vi "Leviathan_Main_v4.1.0.vi"() -> ()   [LabVIEW 2025]
doc: "In that day, the Lord will punish with his sword - his fierce, great and powerful sword - Leviathan the gliding serpent, Leviathan the coiling serpent; he will slay the monster of the sea.\n-Isaiah 27:1"
uses:
  <vilib>/DAQmx/read.llb/DAQmx Read (Analog 2D DBL NChan NSamp).vi
  94cf692e-9ffa-4bb0-948f-941e7388c268.vi
  9a7535df-366d-4375-9b4f-c4f5a7296935.vi
  <vilib>/DAQmx/write.llb/DAQmx Write (Analog 1D Wfm NChan NSamp).vi
  89056647-3b37-41a7-a948-164930831248.vi
  <vilib>/DAQmx/miscellaneous.llb/DAQmx Fill In Error Info.vi
panel:
  out "Femto Gain V/A":dbl
  in  "Femto Gain V/A":dbl(ring) items=["1E3"=1.0, "1E4"=2.0, "1E5"=3.0, "1E6"=4.0, "1E7"=5.0, "1E8"=6.0, "1E9"=7.0]
  in  "Ch Swap Delay / ms":dbl=50.0 format="%0.0f"
  in  "RESET":bool
  out "# saved":i32
  out "Piezo V":dbl format="%_5g"
  out "Crashed?":bool
  out "G / G0":dbl
  in  "PID ON?":bool
  out "OffGuide":dbl(graph)
  in  "Reset2D":bool
  in  "Reset1D":bool
  in  "RT Analysis ON?":bool
  in  "SAVE?":bool
  out "2D Hist":dbl[][](graph)
  out "RT Bias num / V":dbl
  out "RT Femto num / V":dbl format="%#_3g"
  out "Piezo (V)":dbl(slide) scale=-7.0..7.0
  out "Hist":i32[](graph)
  out "Log(G/G0)":dbl[](graph)
  out "RT Signal":T1(graph)
  in  "Selector":T2(tab)
  in  "PID gains":T3={"proportional gain (Kc)"=-0.01, "integral time (Ti, min)"=9.999999999999982e-05, "derivative time (Td, min)"=0.0} {"derivative time (Td, min)" format="%.6f"; "integral time (Ti, min)" format="%.6f"; "proportional gain (Kc)" format="%.6f"}
  in  "SP Femto / V":dbl=0.1
  out "PID Runtime / s":dbl
  in  "Pulse Bias / V":dbl
  in  "PM wave shape":dbl(ring) items=["triangle", "square", "sine"]
  in  "PM amplitude / nm":dbl
  in  "No of Piezo Modulations per step":dbl
  out "Ramp Time / s":dbl
  in  "Ramp?":bool
  in  "Rp Hgt":dbl=10.0 caption="Ramp Height / nm"
  in  "Ramp Time (1) /s":dbl=1.0
  in  "Offset (0) / nm":dbl min=-200.0 max=200.0 step=1.0 format="%.1g"
  in  "Ramp Select":u16(ring) caption="Ramp Type" items=["Linear Ramp", "Advanced Ramps"]
  in  "Exp Typ":u16(ring) caption="Adv BJ Measurement Method" items=["Piezo Hold", "Square Bias", "Sine Bias", "Triangle Bias", "IV", "PM", "IV - Polarity Sweep", "CV - 2 Terminal", "Pre/Post Pulse IVs WIP"]
  in  "Bias Amp / V":dbl=1.0 caption="Bias Amplitude / V"
  in  "dZ / nm":dbl=1.0 caption="Step Height / nm"
  in  "Steps":i32=10 caption="No of Steps"
  in  "Bias f / Hz":dbl=100.0 caption="Bias modulation frequency / Hz"
  in  "Modulation hold time (0.01) / s":dbl=0.01
  in  "Sharpening Time /s (1) /s":dbl=1.0
  in  "sharpening depth /nm":dbl=50.0
  in  "#Traces/Sharpen":i32=200
  in  "Minimum Log(G/G0)":dbl=-6.0
  in  "Minimum Piezo / nm":dbl=-0.25
  in  "Maximum Log(G/G0)":dbl=0.5
  in  "Maximum Piezo / nm":dbl=3.2
  in  "Upper Bound":dbl=0.5
  in  "Lower Bound":dbl=-5.0
  in  "G0 alignement":dbl=-0.5
  in  "2DHist Intensity":dbl(slide)=101.26582278481013 scale=0.0..3000.0
  out "Ramps":dbl[][](graph)
  in  "Offset (0) / 1E-5":dbl
  in  "Piezo Sensitivity / nm V-1":dbl=1.95
  in  "File Path":path
  in  "Aq Rt (20000) / Hz":dbl=20000.0 format="%0.0f"
  out "Acquire":bool
  in  "DC Bias (0.2) / V":dbl=0.2 format="%_4g"
  # "Leviathan v4.1.0\nJames M. F. Morris | R. Tom Abram | Chiara E. Spano | Roberto Listo | Adam Larbi | Zoë Irlam | Andrea Vezzoli"
  # "Controls:\n\nPg Up - increase offset by 1nm\nHome - Decrease offset by 1 nm\nInsert - Start/Stop Saving\nDelete - Start/Stop PID\nEnd - Start/Stop Ramp\nPg Down - Start/Stop Real time analysis\n\nSaving formatting change:\nDO NOT include a file extension when choosing a \nfile name (e.g. use Directory\\James\\SaveFile NOT Directory\\James\\SaveFile.txt)\n\nPID Info:\nTurning the PID off and leaving the Ramp engaged will activate manual ('James')\nmode.\n\nNOTES:\nThe RESET buttons have a bug, they need to be held down for them to work. Working on fixing this."
  # "NOTES:\n\nPIEZO OSCILATION SETTINGS:\nOscilation frequency calculation:\n\nHold Time = Ramp time / No of steps (units: seconds)\nT  = Hold Time - DC Time (units: seconds)\nOscilation Frequency = No of Piezo Modulations / T (units: hertz)\n\nOscilation amplitude = 2 * PM amplitude (units: nanometers)"
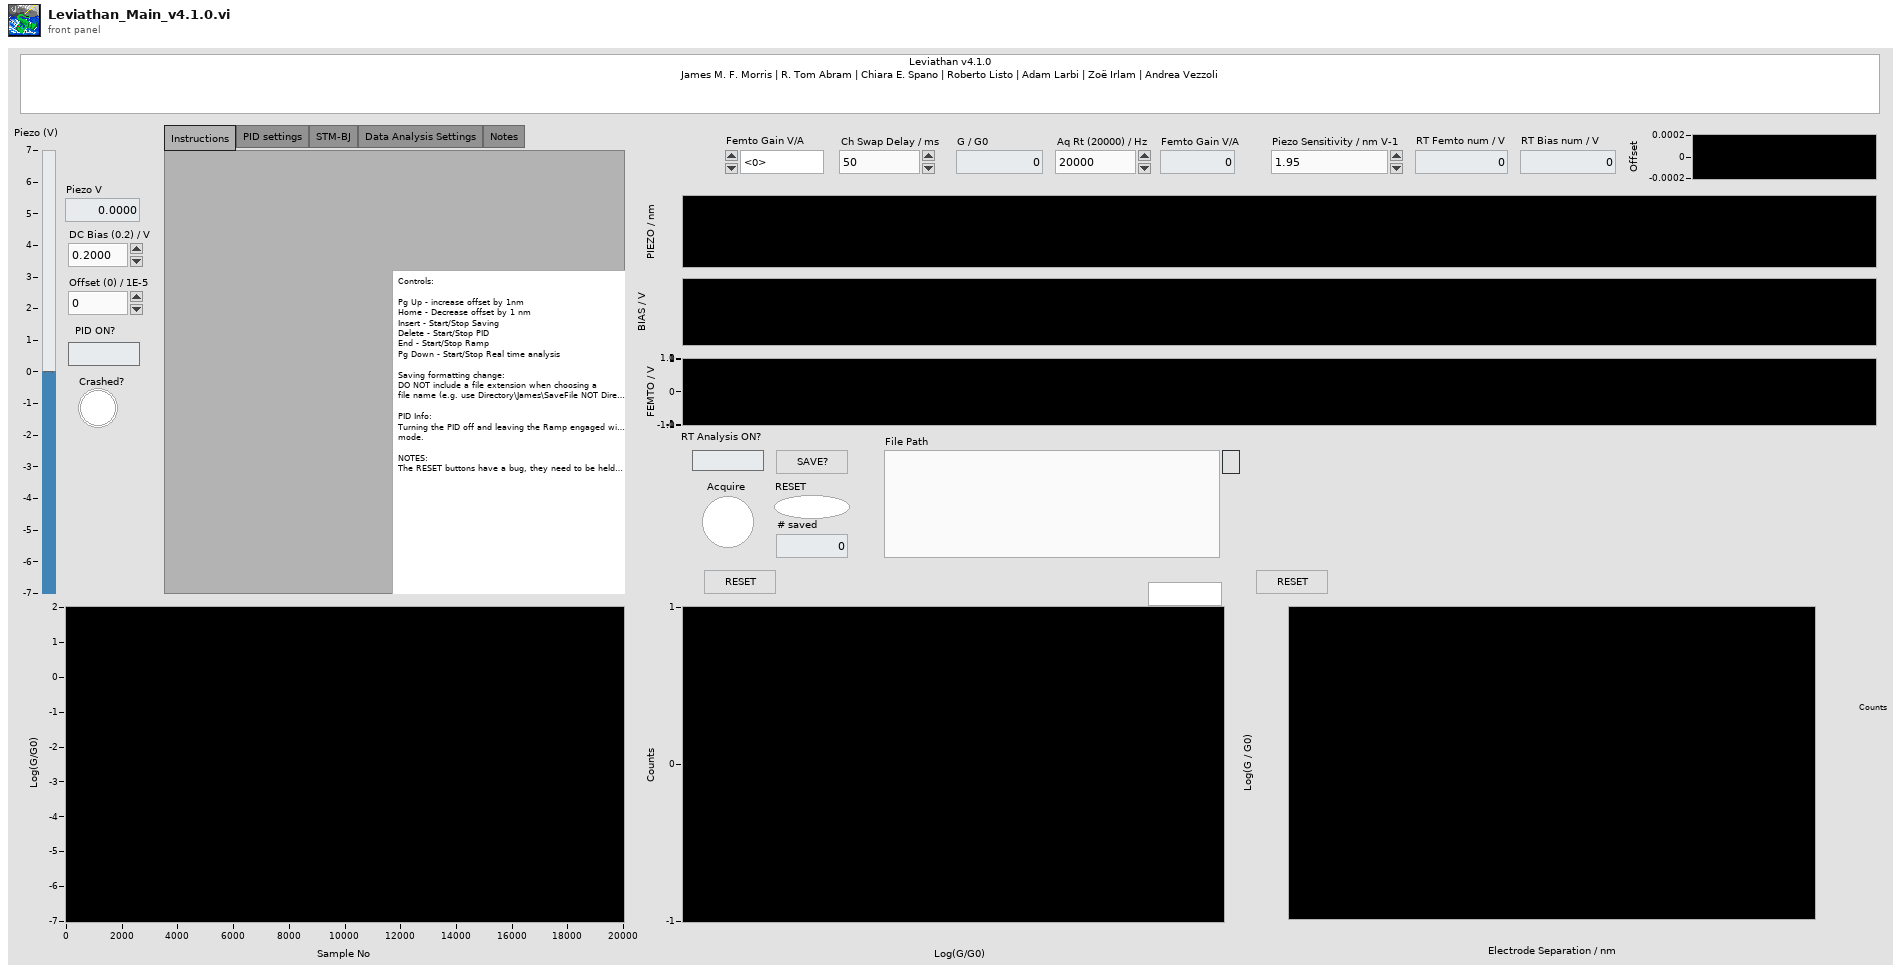
[diagram p1: front panel]
types:
  T1 = cluster{"Piezo / nm":dbl, "Bias / V":dbl, "Real Time Femto /V":dbl}
  T2 = enum32{"Instructions", "PID settings", "STM-BJ", "Data Analysis Settings", "Notes"}
  T3 = cluster{"proportional gain (Kc)":dbl, "integral time (Ti, min)":dbl, "derivative time (Td, min)":dbl}
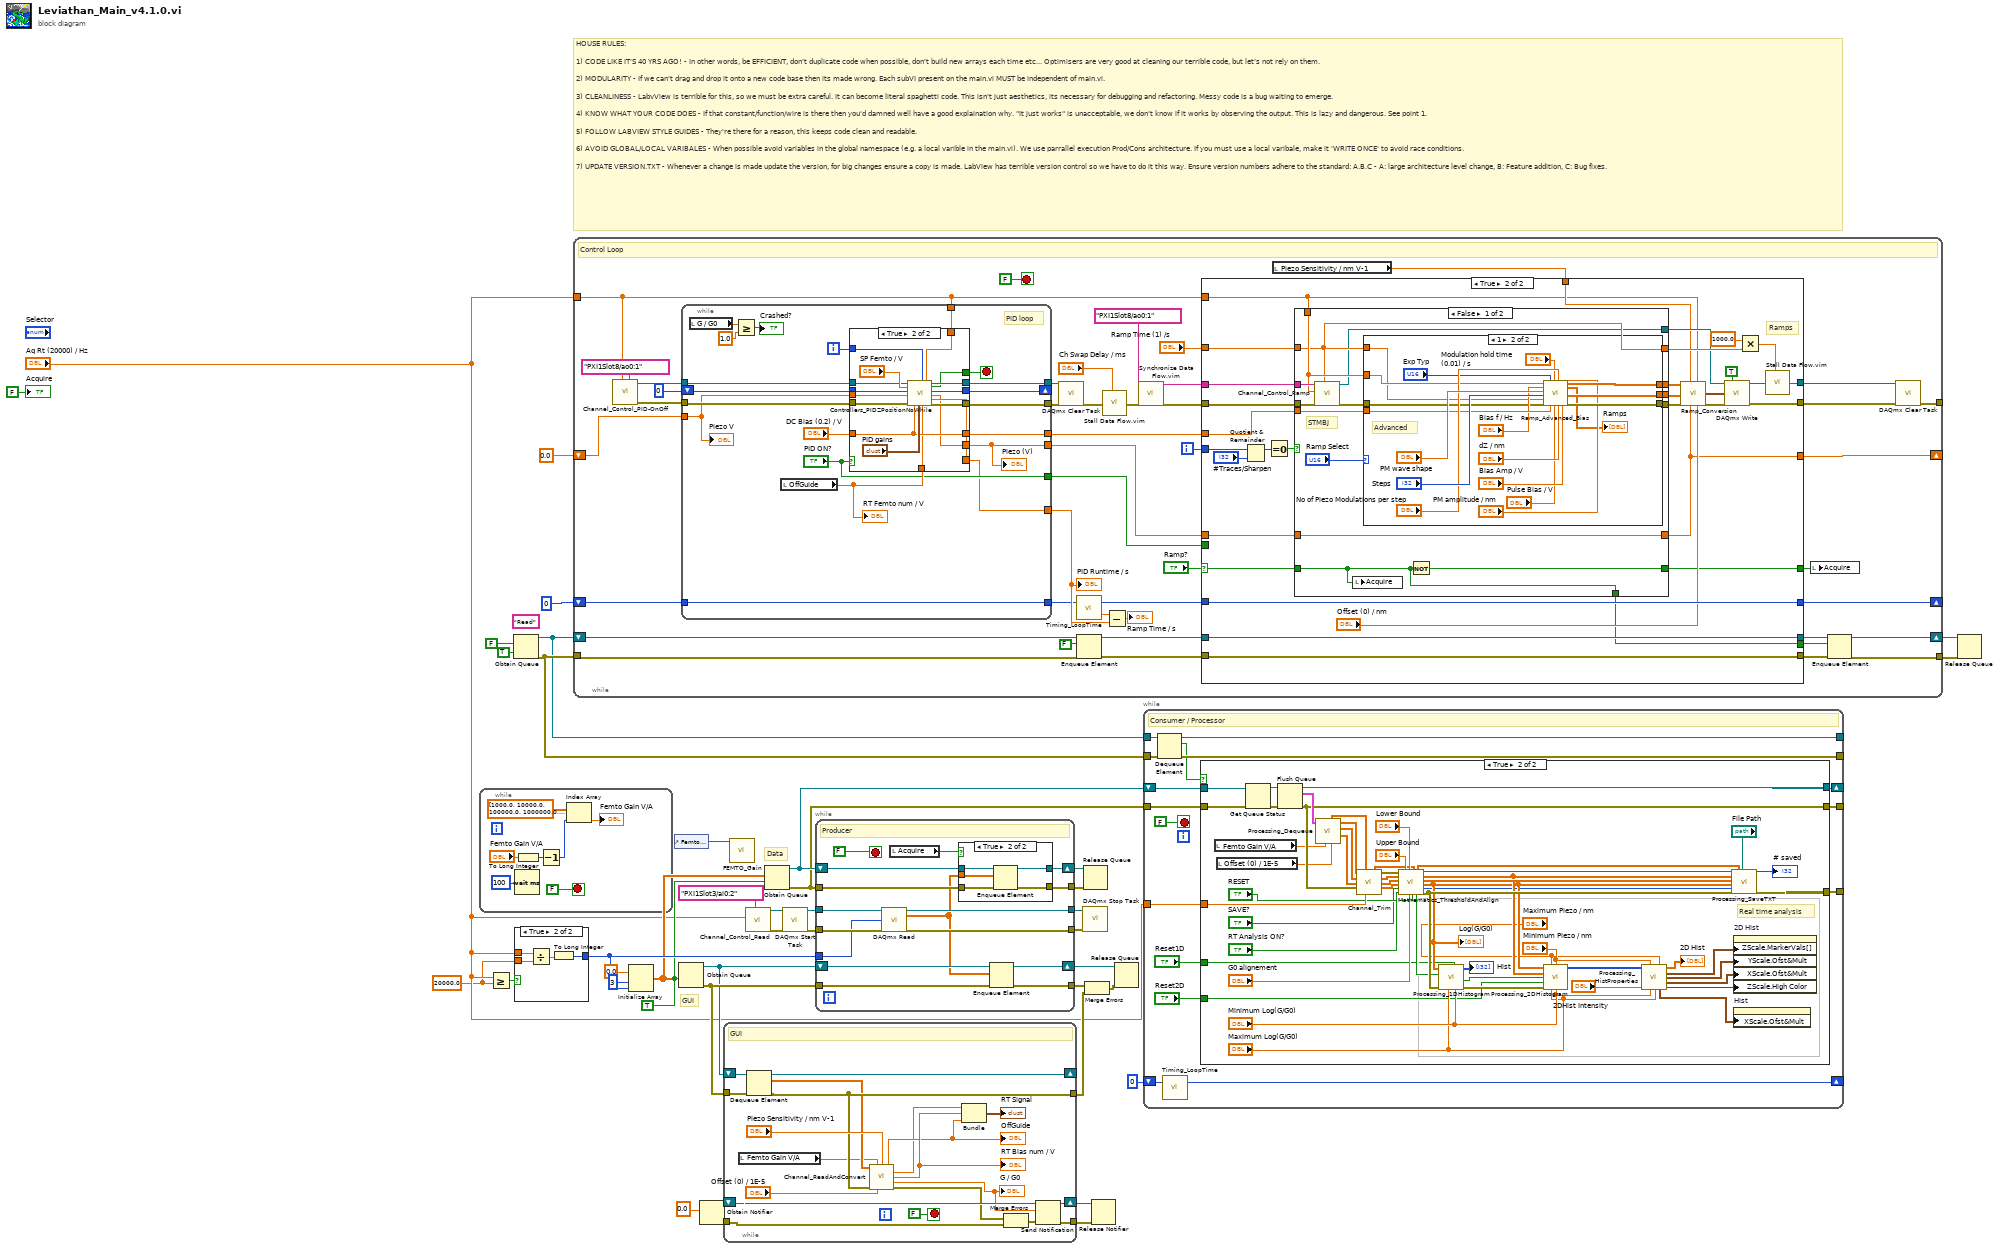
[diagram p0: block diagram]
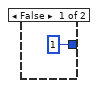
[diagram p2: hidden frame]
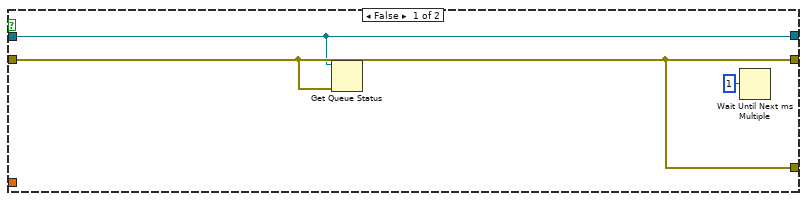
[diagram p4: hidden frame]
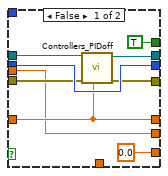
[diagram p5: hidden frame]
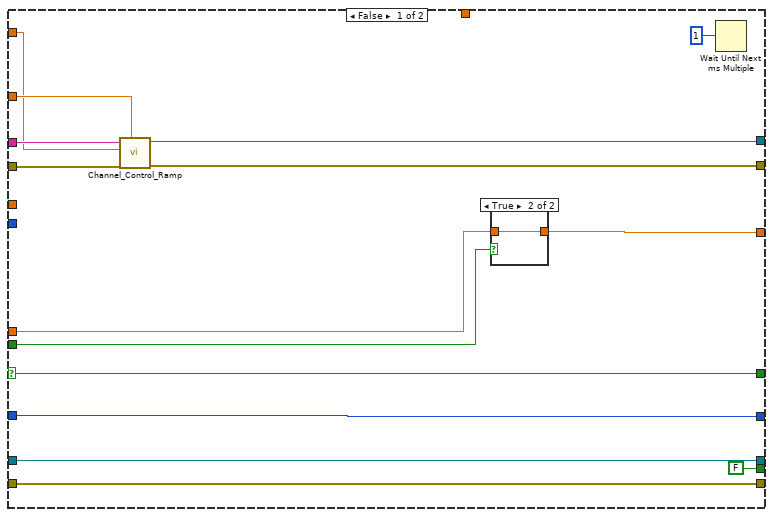
[diagram p6: hidden frame]
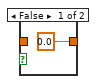
[diagram p7: hidden frame]
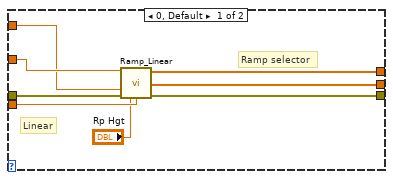
[diagram p8: hidden frame]
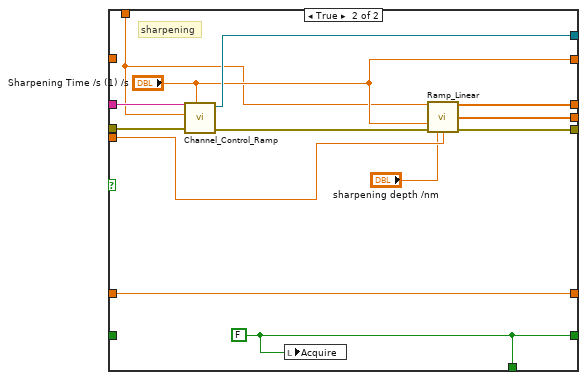
[diagram p9: hidden frame]
diagram:
  w1 = 20000.0 ("y")
  w21 = TRUE ("create if not found? (T)")
  (unwired) "Read" ("name (unnamed)")
  # "Data"
  # "GUI"
  # "HOUSE RULES:\n\n1) CODE LIKE IT'S 40 YRS AGO! - In other words, be EFFICIENT, don't duplicate code when possible, don't build new arrays each time etc... Optimisers are very good at cleaning our terrible code, but let's not rely on them.\n\n2) MODULARITY - If we can't drag and drop it onto a new code base then its made wrong. Each subVI present on the main.vi MUST be independent of main.vi.\n\n3) CLEANLINESS - LabvView is terrible for this, so we must be extra careful. It can become literal spaghetti code. This isn't just aesthetics, its necessary for debugging and refactoring. Messy code is a bug waiting to emerge.\n\n4) KNOW WHAT YOUR CODE DOES - If that constant/function/wire is there then you'd damned well have a good explaination why. \"It just works\" is unacceptable, we don't know if it works by observing the output. This is lazy and dangerous. See point 1.\n\n5) FOLLOW LABVIEW STYLE GUIDES - They're there for a reason, this keeps code clean and readable.\n\n6) AVOID GLOBAL/LOCAL VARIBALES - When possible avoid variables in the global namespace (e.g. a local varible in the main.vi). We use parrallel execution Prod/Cons architecture. If you must use a local varibale, make it 'WRITE ONCE' to avoid race conditions.\n\n7) UPDATE VERSION.TXT - Whenever a change is made update the version, for big changes ensure a copy is made. LabView has terrible version control so we have to do it this way. Ensure version numbers adhere to the standard: A.B.C - A: large architecture level change, B: Feature addition, C: Bug fixes."
  n1 = while {
    stop <- FALSE stop-if-true
    n2 = Wait (ms)(milliseconds to wait=u32 100) -> ()  [unwired: 1 out]
    n3 = To Long Integer(number="Femto Gain V/A") -> (32bit integer=w45:i32)
    n4 = Decrement(x=w45) -> (x-1=w43:i32)
    n5 = Index Array(array=dbl[] [1000.0, 10000.0, 100000.0, 1000000.0, 10000000.0, 100000000.0, 1000000000.0] ("Femto Out / V"), index=w43) -> (element=→"Femto Gain V/A":dbl)
  }
  n6 = Greater Or Equal?(x="Aq Rt (20000) / Hz", y=w1) -> (x >= y?=w3:bool)
  n7 = Obtain Queue(element data type=FALSE ("create if not found? (T)"), create if not found? (T)=TRUE) -> (queue out=w34:refnum<queue>, error out=w35:errorcluster)  [unwired: 3 in, 1 out]
  n8 = case shown="True" w3 {
    tunnel: "Aq Rt (20000) / Hz" -> [_ w53]
    tunnel: [1 w51] -> w22
    tunnel: w1 -> [_ w50]
    frame False {
    }
    frame True {
      n9 = Divide(x=w53, y=w50) -> (x/y=w52:dbl)
      n10 = To Long Integer(number=w52) -> (32bit integer=w51:i32)
    }
  }
  n11 = while {
    shift-right: [w86] -> _
    shift-left: u32 0 ("millisecond timer value") -> [w92]
    tunnel: "Aq Rt (20000) / Hz" -> [w63]
    tunnel: w35 -> [w78]
    shift-right: [w81] -> w37
    shift-left: w34 -> [w77]
    tunnel: [w79] -> w36
    tunnel: [w73] -> _
    shift-right: [w69] -> _
    shift-left: 0.0 ("Piezo Out / V") -> [w68]
    i -> [w65]
    stop <- FALSE stop-if-true
    # "Control Loop"
    n12 = call "Channel_Control_PID-OnOff.vi"("Output Channel PIDonoff"=tag "PXI1Slot8/ao0:1" ("physical channels"), "Aquisition rate / Hz"=w63) -> ("Error Out"=w74:errorcluster, "WRITE PIDonoff"=w72:refnum<k21>)  [unwired: 8 in]
    n13 = while {
      tunnel: [w117] -> w60
      tunnel: [w116] -> w59
      tunnel: w74 -> [w109]
      shift-right: [w115] -> _
      shift-left: u32 0 ("Loop Time Out") -> [w114]
      tunnel: [w99] -> w93
      tunnel: [w98] -> w95
      tunnel: w92 -> [w113]
      tunnel: [w113] -> w91
      tunnel: [w110] -> w90
      tunnel: w63 -> [w108]
      tunnel: w72 -> [w103]
      tunnel: w68 -> [w101]
      tunnel: ["PID ON?"] -> w66
      i -> [w111]
      stop <- w104 stop-if-true
      # "PID loop"
      n14 = local read "G / G0"() -> (w107:dbl)
      n15 = Greater Or Equal?(x=w107, y=1.0) -> (x >= y?=→"Crashed?":bool)
      n16 = local read "OffGuide"() -> (w102:dbl)
      "RT Femto num / V" <- w102
      n17 = case shown="True" "PID ON?" {
        tunnel: [w120 w142] -> w117
        tunnel: [w123 w141] -> w116
        tunnel: w109 -> [w124 w140]
        tunnel: w103 -> [w121 w128]
        tunnel: [w125 w139] -> w115
        tunnel: w114 -> [w125 w138]
        tunnel: [w118 w130] -> w98
        tunnel: "DC Bias (0.2) / V" -> [w122 w131]
        tunnel: [TRUE ("Stop?") w136] -> w104
        tunnel: [0.0 ("Runtime / s") w134] -> w99
        tunnel: w101 -> [w118 w132]
        tunnel: w111 -> [_ w133]
        tunnel: [w122 w131] -> w110
        tunnel: w102 -> [_ w127]
        tunnel: w108 -> [_ w129]
        frame False {
          n18 = call "Controllers_PIDoff.vi"("DC Bias"=w122, "Error In"=w124, "Task in"=w121) -> ("Error Out"=w123:errorcluster, "Task Out"=w120:refnum<k21>)  [unwired: 7 in]
        }
        frame True {
          n19 = call "Controllers_PIDZPositionNoWhile.vi"("Task In"=w128, "SP Femto"="SP Femto / V", "Loop Time In"=w138, "Piezo In / V"=w132, "Error In"=w140, "DC Bias"=w131, "PID gains"="PID gains", "Iterator In"=w133, "Real time Femto / V"=w127, "Aquisition Rate (20000) / Hz"=w129) -> ("Task Out"=w142:refnum<k21>, "Stop?"=w136:bool, "Loop Time Out"=w139:u32, "Piezo Out / V"=w130:dbl, "Runtime / s"=w134:dbl, "Error Out"=w141:errorcluster)  [unwired: 4 in]
        }
      }
      "Piezo (V)" <- w98
      "Piezo V" <- w101
    }
    "PID Runtime / s" <- w93
    n20 = call <vilib>:"DAQmx Clear Task.vi"("task in"=w60, "error in"=w59) -> ("error out"=w56:errorcluster)  [unwired: 13 in]
    n21 = call "Timing_LoopTime.vi"("Loop Time In"=w91) -> ("Runtime / s"=w94:dbl, "Loop Time Out"=w87:u32)  [unwired: 1 in]
    n22 = Enqueue Element(queue=w77, element=FALSE (".not. x?"), error in (no error)=w78) -> (queue out=w85:refnum<queue>, error out=w84:errorcluster)  [unwired: 1 in, 1 out]
    n23 = call "Stall Data Flow.vim"("value in"=w56, "milliseconds to wait"="Ch Swap Delay / ms") -> ("value out"=w55:errorcluster)  [unwired: 1 out]
    n24 = Subtract(x=w94, y=w93) -> (x-y=→"Ramp Time / s":dbl)
    n25 = call "Synchronize Data Flow.vim"("input 4"=w55, "input 1"=tag "PXI1Slot8/ao0:1" ("physical channels")) -> ("output 4"=w61:errorcluster, "output 1"=w62:tag)  [unwired: 2 in, 2 out]
    n26 = local read "Piezo Sensitivity / nm V-1"() -> (w89:dbl)
    n27 = case shown="True" "Ramp?" {
      selector: "Ramp?" -> [w157 w170]
      tunnel: [w146 w191] -> w57
      tunnel: [w145 w184] -> w58
      tunnel: w95 -> [w150 w172]
      tunnel: [w151 w171] -> w69
      tunnel: [w157 w169] -> w88
      tunnel: w90 -> [_ w189]
      tunnel: w89 -> [_ w164]
      tunnel: w87 -> [w155 w188]
      tunnel: [w155 w188] -> w86
      tunnel: w84 -> [w153 w186]
      tunnel: w85 -> [w154 w187]
      tunnel: [w154 w187] -> w82
      tunnel: [w153 w186] -> w80
      tunnel: [FALSE (".not. x?") w161] -> w76
      tunnel: "Ramp Time (1) /s" -> [w144 w181]
      tunnel: w66 -> [w149 _]
      tunnel: w65 -> [_ w173]
      tunnel: w61 -> [w147 w167]
      tunnel: w62 -> [w148 w166]
      tunnel: w63 -> [w143 w160]
      frame False {
        n28 = call "Channel_Control_Ramp.vi"("Ramp Time / s"=w144, "Error In"=w147, "Aquisition rate/ Hz"=w143, "Output Chnnel Ramp"=w148) -> ("Error Out"=w146:errorcluster, "WRITE RAMP"=w145:refnum<k21>)  [unwired: 6 in]
        n29 = case shown="True" w149 {
          tunnel: [0.0 ("Piezo Out / V") w159] -> w151
          tunnel: w150 -> [_ w159]
          frame False {
          }
          frame True {
          }
        }
        n30 = Wait Until Next ms Multiple(millisecond multiple=u32 1 ("milliseconds to wait")) -> ()  [unwired: 1 out]
      }
      frame True {
        # "Ramps"
        n31 = Quotient & Remainder(x=w173, y="#Traces/Sharpen") -> (x-y*floor(x/y)=w162:i32)  [unwired: 1 out]
        n32 = Equal To 0?(x=w162) -> (x = 0?=w163:bool)
        n33 = case shown="False" w163 {
          tunnel: w189 -> [w205 w241]
          tunnel: w160 -> [w196 w234]
          tunnel: w181 -> [w195 _]
          tunnel: [w204 w244] -> w180
          tunnel: [w203 w243] -> w178
          tunnel: [w202 w242] -> w177
          tunnel: w172 -> [w200 w240]
          tunnel: [w200 w240] -> w171
          tunnel: w170 -> [w192 _]
          tunnel: [w199 w233] -> w169
          tunnel: [w195 "Sharpening Time /s (1) /s"] -> w168
          tunnel: w167 -> [w197 w239]
          tunnel: w166 -> [w198 w238]
          tunnel: [w193 w236] -> w165
          tunnel: [w192 w233] -> w161
          frame False {
            # "STMBJ"
            n34 = call "Channel_Control_Ramp.vi"("Ramp Time / s"=w195, "Error In"=w197, "Aquisition rate/ Hz"=w196, "Output Chnnel Ramp"=w198) -> ("Error Out"=w194:errorcluster, "WRITE RAMP"=w193:refnum<k21>)  [unwired: 6 in]
            n35 = local write "Acquire"(w192) -> ()
            n36 = case shown="1" "Ramp Select" {
              tunnel: w205 -> [w213 w224]
              tunnel: w196 -> [w212 w221]
              tunnel: w195 -> [w211 w220]
              tunnel: [w210 w231] -> w204
              tunnel: [w209 w230] -> w203
              tunnel: [w208 w229] -> w202
              tunnel: w194 -> [w207 w216]
              frame 0, Default {
                # "Linear"
                # "Ramp selector"
                n37 = call "Ramp_Linear.vi"("Acquisition Rate (20000) / Hz"=w212, "Ramp Time (1) /s"=w211, "Error in"=w207, "Ramp Height (10) / nm"="Rp Hgt", "DC Bias (0.2) / V"=w213) -> ("Piezo Ramp Out / nm"=w209:dbl[], "Bias Ramp Out / V"=w208:dbl[], "Error Out"=w210:errorcluster)  [unwired: 8 in]
              }
              frame 1 {
                # "Advanced"
                n38 = call "Ramp_Advanced_Bias.vi"("Sampling frequency (20000) / Hz"=w221, "Bias Modulation Frequency (100) / Hz"="Bias f / Hz", "PM wave shape"="PM wave shape", "# Steps (10)"="Steps", "Ramp Time (1) / s"=w220, "Error In"=w216, "Measurement Type / bias"="Exp Typ", "DC Bias (0.2) / V"=w224, "DC time (0.02) / s"="Modulation hold time (0.01) / s", "Pulse Bias / V"="Pulse Bias / V", "Piezo Modulation freq."="No of Piezo Modulations per step", "Step Height (1) / nm"="dZ / nm", "PM compression legnth / nm"="PM amplitude / nm", "Bias Ramp Amplitude (1) / V"="Bias Amp / V") -> ("Piezo Out / nm"=w230:dbl[], "Waveform Graph"=→"Ramps":dbl[][], "Bias Ramp Out / V"=w229:dbl[], "Error Out"=w231:errorcluster)  [unwired: 2 in]
              }
            }
            n39 = Not(x=w192) -> (.not. x?=w199:bool)
          }
          frame True {
            w233 = FALSE
            # "sharpening"
            n40 = call "Channel_Control_Ramp.vi"("Ramp Time / s"="Sharpening Time /s (1) /s", "Error In"=w239, "Aquisition rate/ Hz"=w234, "Output Chnnel Ramp"=w238) -> ("Error Out"=w237:errorcluster, "WRITE RAMP"=w236:refnum<k21>)  [unwired: 6 in]
            n41 = local write "Acquire"(w233) -> ()
            n42 = call "Ramp_Linear.vi"("Acquisition Rate (20000) / Hz"=w234, "Ramp Time (1) /s"="Sharpening Time /s (1) /s", "Error in"=w237, "Ramp Height (10) / nm"="sharpening depth /nm", "DC Bias (0.2) / V"=w241) -> ("Piezo Ramp Out / nm"=w243:dbl[], "Bias Ramp Out / V"=w242:dbl[], "Error Out"=w244:errorcluster)  [unwired: 8 in]
          }
        }
        n43 = call "Ramp_Conversion.vi"("Offset (0) / nm"="Offset (0) / nm", "Sampling rate (20k) / Hz"=w160, "Piezo In (0) / V"=w171, "Piezo Sensitivity (1.95) / nm V-1"=w164, "Error in"=w180, "Bias Ramp In (0) / V"=w177, "Piezo Ramp In (0) / V"=w178) -> ("Error Out"=w179:errorcluster, "appended array"=w176:waveform(dbl)[])  [unwired: 3 in]
        n44 = call-poly <vilib>:"DAQmx Write.vi"("task/channels in"=w165, "auto start"=TRUE, "data"=w176, "error in"=w179) -> ("task out"=w185:refnum<k21>, "error out"=w191:errorcluster)  [unwired: 9 in, 1 out]
        n45 = Multiply(x=1000.0, y=w168) -> (x*y=w182:dbl)
        n46 = call "Stall Data Flow.vim"("value in"=w185, "milliseconds to wait"=w182) -> ("value out"=w184:refnum<k21>)  [unwired: 1 out]
      }
    }
    n47 = local write "Acquire"(w88) -> ()
    n48 = Enqueue Element(queue=w82, element=w76, error in (no error)=w80) -> (queue out=w81:refnum<queue>, error out=w79:errorcluster)  [unwired: 1 in, 1 out]
    n49 = call <vilib>:"DAQmx Clear Task.vi"("task in"=w58, "error in"=w57) -> ("error out"=w73:errorcluster)  [unwired: 13 in]
  }
  n50 = Initialize Array(0.0 ("element"), 3 ("dimension size"), w22) -> (w20:dbl[][])
  n51 = control-ref of="Femto Gain V/A"() -> (w4:refnum<vi>)
  n52 = Obtain Queue(element data type=w20, create if not found? (T)=w21) -> (queue out=w9:refnum<queue>, error out=w10:errorcluster)  [unwired: 3 in, 1 out]
  n53 = Obtain Notifier(notification data type=0.0 ("element")) -> (notifier out=w17:refnum<notifier>, error out=w16:errorcluster)  [unwired: 3 in, 1 out]
  n54 = while {
    tunnel: w16 -> [w253]
    shift-right: [w256] -> w13
    shift-left: w17 -> [w257]
    tunnel: [w255] -> w14
    tunnel: w10 -> [w251]
    tunnel: [w248] -> w7
    shift-right: [w249] -> _
    shift-left: w9 -> [w250]
    stop <- FALSE stop-if-true
    # "GUI"
    n55 = local read "Femto Gain V/A"() -> (w245:dbl)
    n56 = Dequeue Element(queue=w250, error in (no error)=w251) -> (queue out=w249:refnum<queue>, element=w247:dbl[][], error out=w248:errorcluster)  [unwired: 1 in, 1 out]
    n57 = call "Channel_ReadAndConvert.vi"("Element In (2D Arr)"=w247, "Amplification (1E6) / V/A"=w245, "Piezo Sensitivity (1.95) / nm V-1"="Piezo Sensitivity / nm V-1", "Error in"=w248, "Offset (0) / 1E-5 V"="Offset (0) / 1E-5") -> ("Real Time Femto /V"=w259:dbl, "Piezo / nm"=w258:dbl, "Bias / V"=w261:dbl, "G / G0"=w246:dbl, "Error Out"=w252:errorcluster)  [unwired: 6 in]
    "RT Bias num / V" <- w261
    "OffGuide" <- w259
    "G / G0" <- w246
    n58 = Bundle("Piezo / nm"=w258, "Bias / V"=w261, "Real Time Femto /V"=w259) -> (→"RT Signal":T1)  [unwired: 1 in]
    n59 = Merge Errors(w252, w253) -> (w254:errorcluster)
    n60 = Send Notification(notification=w246, notifier=w257, error in (no error)=w254) -> (notifier out=w256:refnum<notifier>, error out=w255:errorcluster)
  }
  n61 = call "FEMTO_Gain.vi"("Femto Gain In V/A"=w4) -> ()  [unwired: 10 in]
  n62 = call "Channel_Control_Read.vi"("Input Channel"=tag "PXI1Slot3/ai0:2", "Acquisition Rate (20000)"="Aq Rt (20000) / Hz") -> ("Error Out"=w29:errorcluster, "READ"=w30:refnum<k21>)  [unwired: 8 in]
  n63 = Obtain Queue(element data type=w20, create if not found? (T)=w21) -> (queue out=w12:refnum<queue>, error out=w11:errorcluster)  [unwired: 3 in, 1 out]
  n64 = call <vilib>:"DAQmx Start Task.vi"("task/channels in"=w30, "error in"=w29) -> ("task out"=w26:refnum<k21>, "error out"=w25:errorcluster)  [unwired: 12 in]
  n65 = while {
    tunnel: w25 -> [w280]
    tunnel: w26 -> [w279]
    tunnel: w22 -> [w278]
    tunnel: [w277] -> w28
    tunnel: [w276] -> w27
    tunnel: w10 -> [w274]
    tunnel: w11 -> [w268]
    tunnel: [w272] -> w6
    tunnel: [w267] -> w18
    shift-right: [w273] -> w5
    shift-left: w9 -> [w275]
    shift-right: [w266] -> w19
    shift-left: w12 -> [w269]
    stop <- FALSE stop-if-true
    # "Producer"
    n66 = call-poly <vilib>:"DAQmx Read.vi"("task/channels in"=w279, "number of samples per channel"=w278, "error in"=w280) -> ("task out"=w277:refnum<k21>, "data"=w265:dbl[][], "error out"=w276:errorcluster)  [unwired: 10 in]
    n67 = local read "Acquire"() -> (w270:bool)
    n68 = case shown="True" w270 {
      tunnel: w269 -> [w282 w287]
      tunnel: w268 -> [w281 w286]
      tunnel: [w281 w285] -> w267
      tunnel: [w282 w284] -> w266
      tunnel: w265 -> [_ w283]
      frame False {
      }
      frame True {
        n69 = Enqueue Element(queue=w287, element=w283, error in (no error)=w286) -> (queue out=w284:refnum<queue>, error out=w285:errorcluster)  [unwired: 1 in, 1 out]
      }
    }
    n70 = Enqueue Element(queue=w275, element=w265, error in (no error)=w274) -> (queue out=w273:refnum<queue>, error out=w272:errorcluster)  [unwired: 1 in, 1 out]
  }
  n71 = call <vilib>:"DAQmx Stop Task.vi"("task/channels in"=w28, "error in"=w27) -> ()  [unwired: 12 in, 2 out]
  n72 = Release Queue(queue=w19, error in (no error)=w18) -> ()  [unwired: 1 in, 3 out]
  n73 = Merge Errors(w6, w7) -> (w8:errorcluster)
  n74 = Release Notifier(notifier=w13, error in (no error)=w14) -> ()  [unwired: 1 in, 3 out]
  n75 = Release Queue(queue=w5, error in (no error)=w8) -> ()  [unwired: 1 in, 3 out]
  n76 = while {
    shift-right: [w303] -> _
    shift-left: w12 -> [w291]
    tunnel: w11 -> [w292]
    tunnel: [w302] -> _
    tunnel: [w301] -> _
    shift-right: [w299] -> _
    shift-left: u32 0 ("Loop Time Out") -> [w300]
    tunnel: w34 -> [w298]
    tunnel: w35 -> [w297]
    tunnel: [w296] -> _
    tunnel: [w295] -> _
    tunnel: "Aq Rt (20000) / Hz" -> [w290]
    stop <- FALSE stop-if-true
    # "Consumer / Processor"
    n77 = Dequeue Element(queue=w298, error in (no error)=w297) -> (queue out=w296:refnum<queue>, element=w294:bool, error out=w295:errorcluster)  [unwired: 1 in, 1 out]
    n78 = call "Timing_LoopTime.vi"("Loop Time In"=w300) -> ("Loop Time Out"=w299:u32)  [unwired: 1 in, 1 out]
    n79 = case shown="True" w294 {
      tunnel: w291 -> [w305 w349]
      tunnel: w292 -> [w306 w348]
      tunnel: [w305 w345] -> w303
      tunnel: [w306 w320] -> w302
      tunnel: [w306 w319] -> w301
      tunnel: w290 -> [_ w321]
      tunnel: "Reset1D" -> [_ w318]
      tunnel: "Reset2D" -> [_ w317]
      frame False {
        n80 = Get Queue Status(queue=w305, error in (no error)=w306) -> ()  [unwired: 1 in, 8 out]
        n81 = Wait Until Next ms Multiple(millisecond multiple=u32 1 ("milliseconds to wait")) -> ()  [unwired: 1 out]
      }
      frame True {
        # "Real time analysis"
        n82 = local read "Femto Gain V/A"() -> (w307:dbl)
        n83 = local read "Offset (0) / 1E-5"() -> (w311:dbl)
        n84 = Get Queue Status(queue=w349, error in (no error)=w348) -> (queue out=w347:refnum<queue>, error out=w346:errorcluster)  [unwired: 1 in, 6 out]
        n85 = Flush Queue(queue=w347, error in (no error)=w346) -> (queue out=w345:refnum<queue>, remaining elements=w344:cluster{dbl[][]}[], error out=w320:errorcluster)
        n86 = call "Processing_Dequeue.vi"("Offset (0) / 1E-5"=w311, "Amp (1E6) / V A-1"=w307, "Flushed Elements"=w344) -> ("G / G0"=w341:dbl[], "Bias / V"=w342:dbl[], "Piezo / nm"=w343:dbl[], "Femto / V"=w310:dbl[])  [unwired: 5 in]
        n87 = call "Channel_Trim.vi"("Piezo / nm"=w343, "Femto in / V"=w310, "Bias / V"=w342, "G/G0"=w341, "Error In"=w320, "Aq Rt (20000) / Hz"=w321) -> ("Femto out / V"=w309:dbl[], "Error Out"=w359:errorcluster, "Piezo / nm Trim"=w358:dbl[], "Bias / V Trim"=w357:dbl[], "G/G0 Trim"=w356:dbl[])  [unwired: 5 in]
        n88 = call "Mathematics_ThresholdAndAlign.vi"("Error In"=w359, "Piezo / nm"=w358, "Bias In / V"=w357, "G/G0"=w356, "SAVE?"="SAVE?", "On-The-Fly Data Analysis ON"="RT Analysis ON?", "UP Bound"="Upper Bound", "LOW bound"="Lower Bound", "Alignment Log(G/G0)"="G0 alignement", "Femto In / V"=w309, "RESET"="RESET") -> ("Femto Out / V"=w308:dbl[], "Enable Histograms?"=w352:bool, "Save File?"=w312:bool, "Adj. Piezo / nm"=w340:dbl[], "Bias Out / V"=w355:dbl[], "Log(G/G0)"=w338:dbl[], "#saved files"=w316:u32, "Error Out"=w353:errorcluster)  [unwired: 1 in]
        "Log(G/G0)" <- w338
        n89 = call "Processing_1DHistogram.vi"("Minimum Log(G/G0) (-6)"="Minimum Log(G/G0)", "Reset"=w318, "Maximum Log(G/G0) (0.5)"="Maximum Log(G/G0)", "Error In"=w353, "Enable?"=w352, "Log(G/G0)"=w338) -> ("Error Out"=w350:errorcluster, "Enable? Out"=w351:bool, "Histogram"=→"Hist":i32[])  [unwired: 3 in]
        n90 = call "Processing_2DHistogram.vi"("Log(G/G0)"=w338, "Maximum Piezo / nm"="Maximum Piezo / nm", "Minimum Piezo / nm"="Minimum Piezo / nm", "Piezo / nm"=w340, "Enable?"=w351, "Reset"=w317, "Error In"=w350, "Maximum Log(G/G0)"="Maximum Log(G/G0)", "Minimum Log(G/G0)"="Minimum Log(G/G0)") -> ("Histogram"=w337:i32[][])  [unwired: 5 in, 1 out]
        n91 = call "Processing_HistProperties.vi"("Histogram"=w337, "Minimum Piezo (-0.25) / nm"="Minimum Piezo / nm", "Maximum Piezo (3.2) / nm"="Maximum Piezo / nm", "2D intensity"="2DHist Intensity", "Minimum Log(G/G0) (-6)"="Minimum Log(G/G0)", "Maximum Log(G/G0) (0.5)"="Maximum Log(G/G0)") -> ("Intensity Graph Input"=→"2D Hist":dbl[][], "2DHist-ZScale.MarkerVals[]"=w333:cluster{sgl, u32}[], "2DHist-YScale.Ofst&Mult"=w332:cluster{"Minimum Log(G/G0)":dbl, dbl}, "2DHist-XScale.Ofst&Mult"=w331:cluster{"Minimum Log(G/G0)":dbl, dbl}, "1DHist-XScale.Ofst&Mult"=w329:cluster{"Minimum Log(G/G0)":dbl, dbl}, "2DHist-ZScale.HighColor"=w330:u32)  [unwired: 4 in]
        n92 = call "Processing_SaveTXT.vi"("Save?"=w312, "Piezo/nm"=w340, "Bias/v"=w355, "Log(G/G0)"=w338, "File No"=w316, "Error In"=w353, "Femto / V"=w308, "File Path (use dialog)"="File Path") -> ("File No Out"=→"# saved":i32, "Error Out"=w319:errorcluster)  [unwired: 10 in]
        n93 = property on="2D Hist" class="IntGraph (strict)"("ZScale.MarkerVals[]"=w333, "YScale.Ofst&Mult"=w332, "XScale.Ofst&Mult"=w331, "ZScale.High Color"=w330) -> ()  [unwired: 2 in, 2 out]
        n94 = property on="Hist" class="WFGraph (strict)"("XScale.Ofst&Mult"=w329) -> ()  [unwired: 2 in, 2 out]
      }
    }
  }
  n95 = Release Queue(queue=w37, error in (no error)=w36) -> ()  [unwired: 1 in, 3 out]
  "Acquire" <- FALSE ("Aquire")
